vi "WILT Agilent Read 5 Units.vi"(0 "Agilent Refs":refnum<visa-resource-name>[](array[refnum])=["AGILENT1", "AGILENT2", "AGILENT3", "AGILENT4", "AGILENT5", "AGILENT6", "AGILENT7"], 2 "Data Array":T2, 5 "error in (no error)":errorcluster, 6 "Semaphore":T1[](array[typedef])) -> (14 "Data Out Array":T2, 15 "Uncorrected Agilent Data":dbl[](array[numeric])=[0.0150789, 0.0050262, 0.0083772, 0.0050262, 0.0050262, 0.0067017, 0.0016755, -0.003351, -0.0067017, 0.0050262, 0.0083772, 0.0, 0.0167544, 0.003351, 0.0083772, 0.0117279, 0.0016755, 0.0, 0.0050262, 0.0134034, 0.0067017, 0.0100527, 0.0067017, 0.0117279, 0.0134034, 0.0050262, 0.003351, 0.0016755, 0.0016755, 0.0016755, 0.0134034, -0.0217806, 0.0150789, -0.035184, 0.0, -0.003351, -0.0050262, 0.0134034, 0.0067017, 0.0050262, 3.9473127, 0.0050262, 6.5274765, 0.0268068, 4.0310841, 0.0150789, 0.0050262, 4.2958026, 0.0, 0.0066063, -0.003303, -0.0049545, 0.0148638, 0.0115608, -0.0016515, 0.0148638, 0.0082578, 0.003303, -0.0379854, 0.0, -0.0066063, 4.0198662, 6.30561, 0.003303, -0.429402, 239.21058, 260.33393, 239.35922, 0.776226, 133.99018, -0.759711, 167.76441, 130.80268, 132.75152, 235.8414, 235.67624, 236.03959, 234.25591, -262.90871, -2.295648, 9.9e+37, 2088.531, 350.993, 216.711, 284.45, 15.196, 101.93, 282.933, 13.374, 205.472, 284.335, 2.903, 231.773, 276.053, 11.617, 228.706, 289.836, 58.486, 312.921, 30.474, 151.987, 140.873, 81.461, 75.186, 79.218, 81.617, 239.596, 84.634, 110.282, 90.731, 113.609, 85.502, 243.10926, 239.34635, 234.95629, -1.270377, 0.0132741, 0.0082962, 0.0082962, 0.0033186, 3.983859, 0.0, 0.0116148, 0.0082962, 0.0082962, 3.8677116, 0.0016593, 0.0165924, 0.0099555, -0.0016593, 0.0049776, -0.0082962, 0.0066369, 0.0066369, 0.0066369, 0.0132741, 0.0033186, 0.0165924, 0.0082962, 0.019911, 0.0016593, 0.0082962, 0.0049776, 0.0033186, 0.0016593, 0.0099555, 0.0049776, 0.0099555, 0.0049776, 0.0082962, 0.0099555, 0.0066369, -0.0033186, -0.0082962, 0.0016593, 0.0033186, 0.0033186, 0.0066369, 0.0116148, 0.0149331, 0.0, 0.0149331, 0.0016593, 0.0049776, 88.256, 89.978, 109.447, 80.071, 108.495, 85.221, 87.579, 86.432, 88.657, 87.322, 87.586, 85.354, 86.395, 90.659, 81.787, 82.766, 87.266, 83.934, 83.473, 85.136, 87.507, 84.692, 87.442, 82.836, 237.31969, 236.95648, 237.24073, 237.55657, 235.96159, 0.505338, 9.9e+37, 236.67223, 9.9e+37, 200.03512, 9.9e+37, 237.50919, -220.07392, 2.479311, 3.711069, 0.584295, 236.75119, 200.57204], 16 "Corrected Agilent Data":dbl[](array[numeric])=[0.0150789, 0.0050262, 0.0083772, 0.0050262, 0.0050262, 0.0067017, 0.0016755, -0.003351, -0.0067017, 0.0050262, 0.0083772, 0.0, 0.0167544, 0.003351, 0.0083772, 0.0117279, 0.0016755, 0.0, 0.0050262, 0.0134034, 0.0067017, 0.0100527, 0.0067017, 0.0117279, 0.0134034, 0.0050262, 0.003351, 0.0016755, 0.0016755, 0.0016755, 0.0134034, -0.0217806, 0.0150789, -0.035184, 0.0, -0.003351, -0.0050262, 0.0134034, 0.0067017, 0.0050262, 3.9473127, 0.0050262, 6.5274765, 0.0268068, 4.0310841, 0.0150789, 0.0050262, 4.2958026, 0.0, 0.0066063, -0.003303, -0.0049545, 0.0148638, 0.0115608, -0.0016515, 0.0148638, 0.0082578, 0.003303, -0.0379854, 0.0, -0.0066063, 4.0198662, 6.30561, 0.003303, -0.429402, 239.21058, 260.33393, 239.35922, 0.776226, 133.99018, -0.759711, 167.76441, 130.80268, 132.75152, 235.8414, 235.8414, 235.8414, 235.67624, 235.67624, 235.67624, 236.03959, 236.03959, 236.03959, 234.25591, 234.25591, 234.25591, -262.90871, -2.295648, 9.9e+37, 2088.531, 350.993, 216.711, 284.45, 15.196, 101.93, 282.933, 13.374, 205.472, 284.335, 2.903, 231.773, 276.053, 11.617, 228.706, 289.836, 58.486, 312.921, 30.474, 151.987, 140.873, 81.461, 75.186, 79.218, 81.617, 239.596, 84.634, 110.282, 90.731, 113.609, 85.502, 243.10926, 239.34635, 234.95629, -1.270377, 0.0132741, 0.0082962, 0.0082962, 0.0033186, 3.983859, 0.0, 0.0116148, 0.0082962, 0.0082962, 3.8677116, 0.0016593, 0.0165924, 0.0099555, -0.0016593, 0.0049776, -0.0082962, 0.0066369, 0.0066369, 0.0066369, 0.0132741, 0.0033186, 0.0165924, 0.0082962, 0.019911, 0.0016593, 0.0082962, 0.0049776, 0.0033186, 0.0016593, 0.0099555, 0.0049776, 0.0099555, 0.0049776, 0.0082962, 0.0099555, 0.0066369, -0.0033186, -0.0082962, 0.0016593, 0.0033186, 0.0033186, 0.0066369, 0.0116148, 0.0149331, 0.0, 0.0149331, 0.0016593, 0.0049776, 88.256, 89.978, 109.447, 80.071, 108.495, 85.221, 87.579, 86.432, 88.657, 87.322, 87.586, 85.354, 86.395, 90.659, 81.787, 82.766, 87.266, 83.934, 83.473, 85.136, 87.507, 84.692, 87.442, 82.836, 237.31969, 237.31969, 237.31969, 236.95648, 236.95648, 236.95648, 237.24073, 237.24073, 237.24073, 237.55657, 237.55657, 237.55657, 235.96159, 235.96159, 235.96159, 0.505338, 9.9e+37, 236.67223, 236.67223, 236.67223, 9.9e+37, 200.03512, 9.9e+37, 237.50919, 237.50919, 237.50919, -220.07392, 2.479311, 3.711069, 0.584295, 236.75119, 236.75119, 236.75119, 200.57204], 19 "error out":errorcluster)   [LabVIEW 2016]
uses:
  Type Definitions/WILT Agilent Data Cluster.ctl
  Type Definitions/WILT Agilent Channel Definition.ctl
panel:
  out "Num Agilent Data":i32=230
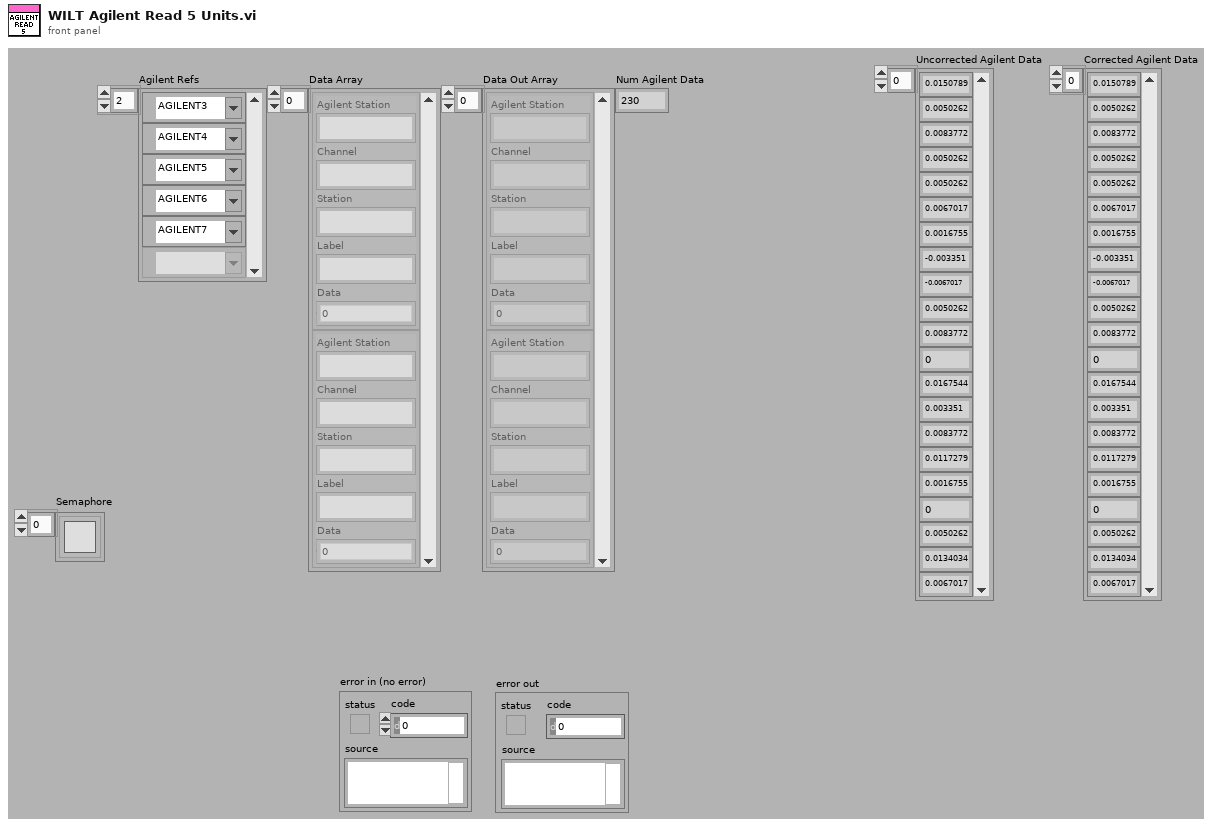
[diagram p1: front panel]
types:
  T1 = typedef "Semaphore RefNum" = refnum<k1>
  T2 = typedef "WILT Agilent Data Cluster.ctl" = T3[]
  T3 = typedef "WILT Agilent Channel Definition.ctl" = cluster{"Channel":string, "Station":string, "Label":string, "Agilent Station":string, "Data":dbl}
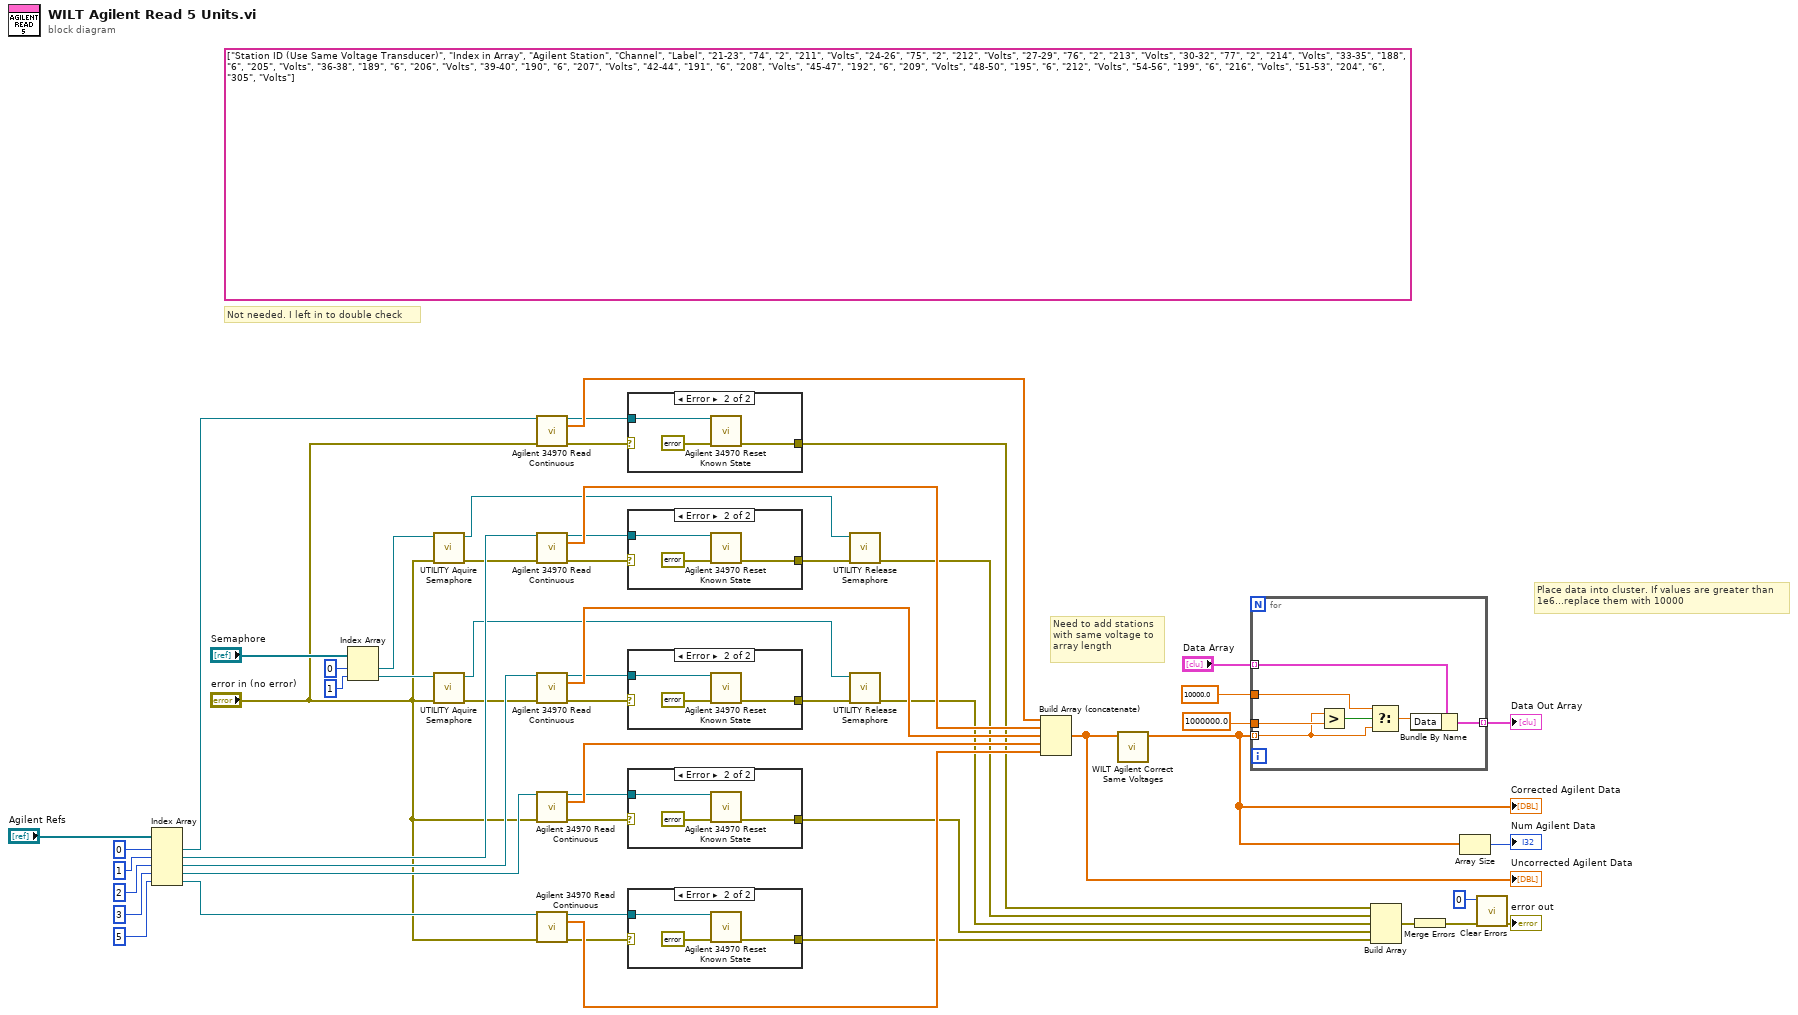
[diagram p0: block diagram]
diagram:
  (unwired) string[][] [["Station ID (Use Same Voltage Transducer)", "Index in Array", "Agilent Station", "Channel", "Label"], ["21-23", "74", "2", "211", "Volts"], ["24-26", "75", "2", "212", "Volts"], ["27-29", "76", "2", "213", "Volts"], ["30-32", "77", "2", "214", "Volts"], ["33-35", "188", "6", "205", "Volts"], ["36-38", "189", "6", "206", "Volts"], ["39-40", "190", "6", "207", "Volts"], ["42-44", "191", "6", "208", "Volts"], ["45-47", "192", "6", "209", "Volts"], ["48-50", "195", "6", "212", "Volts"], ["54-56", "199", "6", "216", "Volts"], ["51-53", "204", "6", "305", "Volts"]] ("Index of stations that use\nthe same voltage")
  # "Not needed. I left in to double check"
  # "Need to add stations\nwith same voltage to\narray length"
  # "Place data into cluster. If values are greater than\n1e6...replace them with 10000"
  n1 = Index Array(array="Agilent Refs", index #1=0 ("index"), index #2=1 ("index"), index #3=2 ("index"), index #4=3 ("index"), index #5=5 ("index")) -> (element #1=w36:refnum<visa-resource-name>, element #2=w35:refnum<visa-resource-name>, element #3=w34:refnum<visa-resource-name>, element #4=w33:refnum<visa-resource-name>, element #5=w32:refnum<visa-resource-name>)
  n2 = Index Array(array="Semaphore", index #1=0, index #2=1) -> (element #1=w26:T1, element #2=w25:T1)
  n3 = call "UTILITY Aquire Semaphore.vi"("error in (no error)"="error in (no error)", "Refnum in"=w26) -> ("error out"=w19:errorcluster, "Refnum out"=w24:T1)  [unwired: 7 in, 1 out]
  n4 = call "UTILITY Aquire Semaphore.vi"("error in (no error)"="error in (no error)", "Refnum in"=w25) -> ("error out"=w18:errorcluster, "Refnum out"=w23:T1)  [unwired: 7 in, 1 out]
  n5 = call "Agilent 34970 Read Continuous.vi"("VISA Resource Name"=w36, "error in (no error)"="error in (no error)") -> ("VISA resource name out"=w10:refnum<visa-resource-name>, "Output Array"=w16:dbl[], "error out"=w12:errorcluster)  [unwired: 10 in, 1 out]
  n6 = call "Agilent 34970 Read Continuous.vi"("VISA Resource Name"=w35, "error in (no error)"=w19) -> ("VISA resource name out"=w13:refnum<visa-resource-name>, "Output Array"=w47:dbl[], "error out"=w15:errorcluster)  [unwired: 10 in, 1 out]
  n7 = call "Agilent 34970 Read Continuous.vi"("VISA Resource Name"=w34, "error in (no error)"=w18) -> ("VISA resource name out"=w7:refnum<visa-resource-name>, "Output Array"=w46:dbl[], "error out"=w9:errorcluster)  [unwired: 10 in, 1 out]
  n8 = call "Agilent 34970 Read Continuous.vi"("VISA Resource Name"=w33, "error in (no error)"="error in (no error)") -> ("VISA resource name out"=w4:refnum<visa-resource-name>, "Output Array"=w45:dbl[], "error out"=w6:errorcluster)  [unwired: 10 in, 1 out]
  n9 = call "Agilent 34970 Read Continuous.vi"("VISA Resource Name"=w32, "error in (no error)"="error in (no error)") -> ("VISA resource name out"=w1:refnum<visa-resource-name>, "Output Array"=w44:dbl[], "error out"=w3:errorcluster)  [unwired: 10 in, 1 out]
  n10 = case shown="Error" w12 {
    selector: w12 -> [w55 _]
    tunnel: [w55 w56] -> w11
    tunnel: w10 -> [_ w57]
    frame No Error {
    }
    frame Error {
      n11 = call "Agilent 34970 Reset Known State.vi"("Error In"=errorcluster {"status"=TRUE, "code"=0, "source"=""}, "VISA Refnum in"=w57) -> ("Error Out"=w56:errorcluster)  [unwired: 9 in]
    }
  }
  n12 = case shown="Error" w15 {
    selector: w15 -> [w59 _]
    tunnel: [w59 w60] -> w14
    tunnel: w13 -> [_ w61]
    frame No Error {
    }
    frame Error {
      n13 = call "Agilent 34970 Reset Known State.vi"("Error In"=errorcluster {"status"=TRUE, "code"=0, "source"=""}, "VISA Refnum in"=w61) -> ("Error Out"=w60:errorcluster)  [unwired: 9 in]
    }
  }
  n14 = case shown="Error" w9 {
    selector: w9 -> [w63 _]
    tunnel: [w63 w64] -> w8
    tunnel: w7 -> [_ w65]
    frame No Error {
    }
    frame Error {
      n15 = call "Agilent 34970 Reset Known State.vi"("Error In"=errorcluster {"status"=TRUE, "code"=0, "source"=""}, "VISA Refnum in"=w65) -> ("Error Out"=w64:errorcluster)  [unwired: 9 in]
    }
  }
  n16 = case shown="Error" w6 {
    selector: w6 -> [w67 _]
    tunnel: [w67 w68] -> w5
    tunnel: w4 -> [_ w69]
    frame No Error {
    }
    frame Error {
      n17 = call "Agilent 34970 Reset Known State.vi"("Error In"=errorcluster {"status"=TRUE, "code"=0, "source"=""}, "VISA Refnum in"=w69) -> ("Error Out"=w68:errorcluster)  [unwired: 9 in]
    }
  }
  n18 = case shown="Error" w3 {
    selector: w3 -> [w71 _]
    tunnel: [w71 w72] -> w2
    tunnel: w1 -> [_ w73]
    frame No Error {
    }
    frame Error {
      n19 = call "Agilent 34970 Reset Known State.vi"("Error In"=errorcluster {"status"=TRUE, "code"=0, "source"=""}, "VISA Refnum in"=w73) -> ("Error Out"=w72:errorcluster)  [unwired: 9 in]
    }
  }
  n20 = call "UTILITY Release Semaphore.vi"("error in (no error)"=w14, "Refnum in"=w24) -> ("error out"=w22:errorcluster)  [unwired: 9 in]
  n21 = call "UTILITY Release Semaphore.vi"("error in (no error)"=w8, "Refnum in"=w23) -> ("error out"=w21:errorcluster)  [unwired: 9 in]
  n22 = Build Array (concatenate)(w16, w47, w46, w45, w44) -> (w39:dbl[])
  "Uncorrected Agilent Data" <- w39
  n23 = call "WILT Agilent Correct Same Voltages.vi"("Standard Agilent Data"=w39) -> ("Corrected Agilent Data"=w38:dbl[])  [unwired: 10 in]
  "Corrected Agilent Data" <- w38
  n24 = for {
    tunnel: "Data Array" -> [w81] mode=indexing
    tunnel: w38 -> [w76] mode=indexing
    tunnel: [w80] -> w42 mode=indexing
    tunnel: 1000000.0 ("y") -> [w79]
    tunnel: 10000.0 ("t") -> [w77]
    n25 = Greater?(x=w76, y=w79) -> (0:w78:bool)
    n26 = Select(t=w77, s=w78, f=w76) -> (s? t:f=w75:dbl)
    n27 = Bundle By Name(cluster=w81, "Data"=w75) -> (w80:T3)
  }
  "Data Out Array" <- w42
  n28 = Build Array(w11, w22, w21, w5, w2) -> (w48:errorcluster[])
  n29 = Merge Errors(w48) -> (w20:errorcluster)
  n30 = Array Size(array=w38) -> (size(s)=→"Num Agilent Data":i32)
  n31 = call <vilib>:"Clear Errors.vi"("error in (no error)"=w20, "specific error code to clear (0: all)"=0) -> ("error out"=→"error out":errorcluster)  [unwired: 4 in, 1 out]
